vi "Configure LINX Device.vi"(5 "Wifi Configuration":T1={"SSID"="", "IP Address"="", "Port"=0, "WIFI Security Type"=enum."WPA2 Password", "Password"=""}, 7 "TCP Configuration":T3, 8 "Error In":errorcluster, 10 "Firmware Interface":T4, 11 "COM Port":refnum<visa-resource-name>) -> (0 "Error Out":errorcluster)   [LabVIEW 2020, in "LMH-LINX.lvlib" / "Device.lvlib"]
uses:
  Device.lvlib
  Type Defs/Firmware Interface.ctl
  Type Defs/TCP Config.ctl
  Type Defs/Wifi Config.ctl
  Type Defs/WIFI Security Type.ctl
  LMH-LINX.lvlib
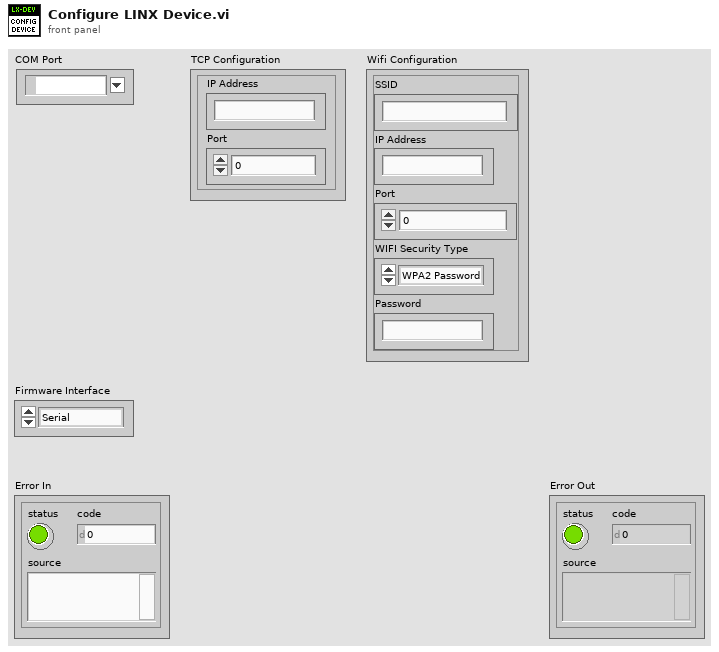
[diagram p1: front panel]
types:
  T1 = typedef "LMH-LINX.lvlib/Device.lvlib/Wifi Config.ctl" = cluster{"SSID":string, "IP Address":string, "Port":u16, "WIFI Security Type":T2, "Password":string}
  T2 = typedef "LMH-LINX.lvlib/WIFI Security Type.ctl" = enum8{"None", "WPA2 Password", "WPA2 Key", "WEP40", "WEP104"}
  T3 = typedef "LMH-LINX.lvlib/Device.lvlib/TCP Config.ctl" = cluster{"IP Address":string, "Port":u16}
  T4 = typedef "LMH-LINX.lvlib/Firmware Interface.ctl" = enum32{"Serial ", "Ethernet", "WIFI"}
  T5 = typedef "LMH-LINX.lvlib/Device.lvlib/LINX Device Config.ctl" = cluster{"Interface":T6, "COM Port":refnum<visa-resource-name>, "TCP Configuration":T3, "Device Family":u8, "Device ID":u8, "Device Name":string, "TCP Ref":refnum<k5>, "Channels":T7}
  T6 = typedef "LMH-LINX.lvlib/Interface.ctl" = enum16{"Serial", "TCP"}
  T7 = typedef "LMH-LINX.lvlib/Channels.ctl" = cluster{"DI":u8[], "DO":u8[], "AI":u8[], "AO":u8[], "PWM":u8[], "QE":u8[], "UART":u8[], "I2C 2":u8[], "SPI":u8[], "CAN":u8[], "Servo":u8[], "AI Ref (V)":dbl, "AI Resolution (Bits)":u8, "AO Ref (V)":dbl, "AO Resolution (Bits)":u8}
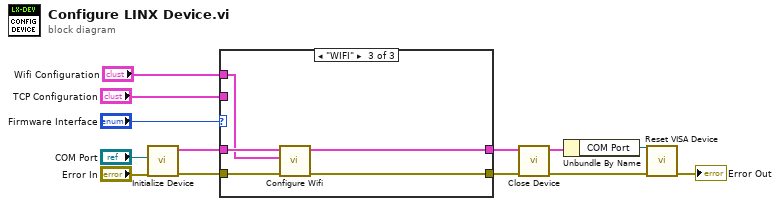
[diagram p0: block diagram]
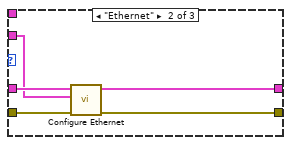
[diagram p3: hidden frame]
diagram:
  n1 = call "Initialize Device.vi"("Error In"="Error In", "COM Port"="COM Port") -> ("Error Out"=w10:errorcluster, "LINX Device Config"=w11:T5)  [unwired: 8 in]
  n2 = case shown="\"WIFI\"" "Firmware Interface" {
    tunnel: w11 -> [w14 w20 w23]
    tunnel: w10 -> [w15 w19 w22]
    tunnel: [w14 w18 w24] -> w4
    tunnel: [w15 w17 w25] -> w3
    tunnel: "TCP Configuration" -> [_ w16 _]
    tunnel: "Wifi Configuration" -> [_ _ w21]
    frame "Serial ", Default {
    }
    frame "Ethernet" {
      n3 = call "Configure Ethernet.vi"("Error In"=w19, "TCP Configuration"=w16, "LINX Device Config"=w20) -> ("Error Out"=w17:errorcluster, "LINX Device Config"=w18:T5)  [unwired: 7 in]
    }
    frame "WIFI" {
      n4 = call "Configure Wifi.vi"("Error In"=w22, "Wifi Configuration"=w21, "LINX Device Config"=w23) -> ("Error Out"=w25:errorcluster, "LINX Device Config"=w24:T5)  [unwired: 7 in]
    }
  }
  n5 = call "Close Device.vi"("Error In"=w3, "LINX Device Config"=w4) -> ("Error Out"=w9:errorcluster, "LINX Device Config"=w8:T5)  [unwired: 8 in]
  n6 = Unbundle By Name(w8) -> ("COM Port"=w7:refnum<visa-resource-name>)
  n7 = call "Reset VISA Device.vi"("Error In"=w9, "VISA resource name"=w7) -> ("Error Out"=→"Error Out":errorcluster)  [unwired: 9 in]
